vi "TestLocalize.vi"() -> ()   [LabVIEW 2011]
uses:
  JTrkAPI.llb/TrackerDLL.vi
panel:
  in  "Use QI":bool=TRUE
  in  "QI iterations":i32=2
  out "error":bool
  out "QI results":cluster{dbl, dbl}(graph)
  in  "ZLUT radius":sgl=32.0
  in  "profileWidth":i32=32
  out "ZLUT":sgl[][](graph)
  out "Intensity Graph":sgl[][](graph)
  in  "image size":cluster{"width":u32, "height":u32}={"width"=150, "height"=150}
  in  "Z random factor":dbl
  in  "z center":dbl=0.5
  out "Z localization":dbl(graph)
  in  "x scalefactor":sgl=0.1
  out "X Chart":dbl(graph)
  in  "jump period":i32=20
  in  "XCorWindow":u32=128
  in  "maxphotoncount":sgl=50000.0
  in  "Max Z":sgl=6.0
  in  "Min Z":sgl=1.0
  in  "Z planes":i32=60
  out "FPS":dbl
  out "Loop count":i32
  out "appended path":path
  in  "Show graphs":bool
  in  "Use debug library":bool
  in  "xcor_iterations":i32=2
  out "X profile":sgl[](graph)
  out "Y profile":sgl[](graph)
  out "Y result":sgl[](graph)
  out "True Y":dbl
  out "True X":dbl
  out "COM results":cluster{dbl, dbl}(graph)
  out "XCor results":cluster{dbl, dbl}(graph)
  in  "y center":dbl=75.0
  in  "x center":dbl=75.0 min=40.0 max=200.0
  out "X result":sgl[](graph)
  in  "Stop loop":bool
  out "median":sgl
  out "xcorpos":cluster{"XCor X":sgl, "XCor Y":sgl}
  out "COM":cluster{"comX":sgl, "comY":sgl}
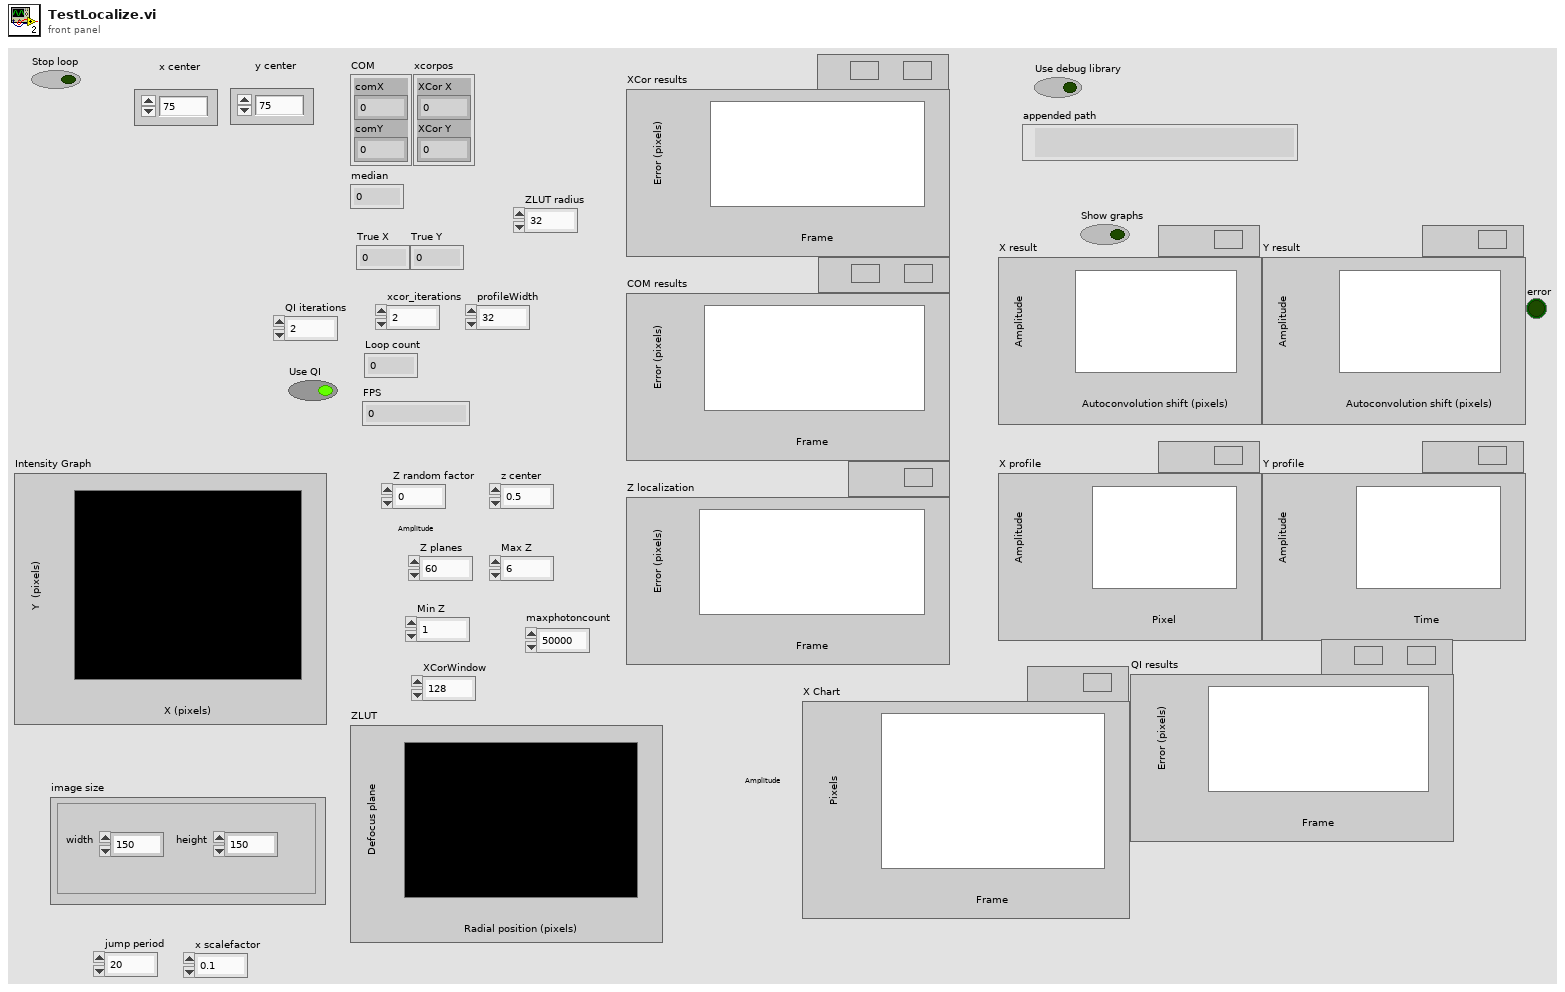
[diagram p1: front panel]
types:
  T1 = typedef "TrackerInstance.ctl" = cluster{"Tracker Pointer":u64, "Image size":cluster{"width":u32, "height":u32}}
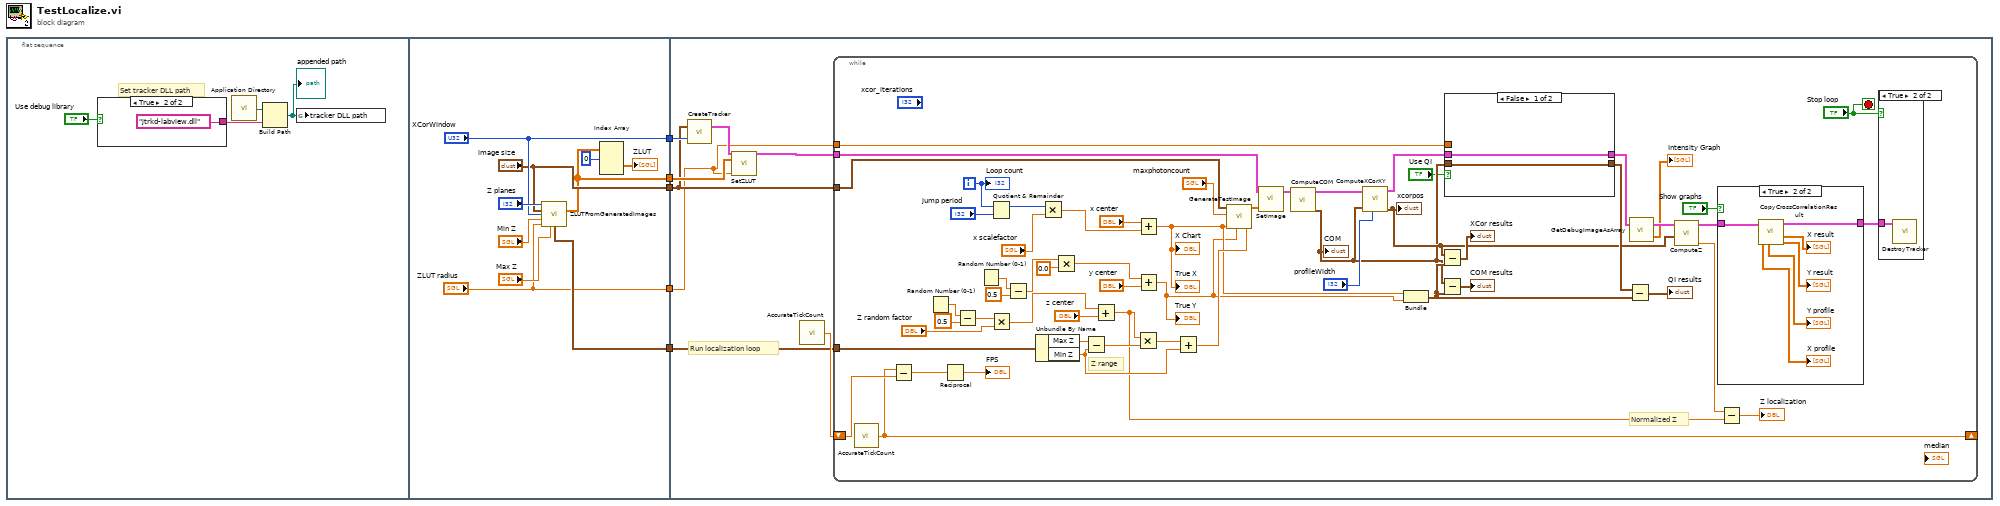
[diagram p0: block diagram]
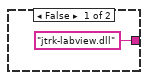
[diagram p2: hidden frame]
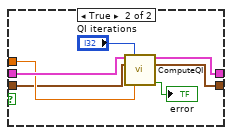
[diagram p3: hidden frame]
diagram:
  n1 = flat-sequence {
    tunnel: [w20] -> w5
    tunnel: ["image size"] -> w4
    tunnel: ["XCorWindow"] -> w3
    tunnel: [w13] -> w2
    tunnel: ["ZLUT radius"] -> w1
    tunnel: w5 -> [w28]
    tunnel: w4 -> [w25]
    tunnel: w3 -> [w27]
    tunnel: w2 -> [w26]
    tunnel: w1 -> [w22]
    frame #0 {
      # "Set tracker DLL path"
      n2 = case shown="True" "Use debug library" {
        tunnel: ["jtrk-labview.dll" "jtrkd-labview.dll"] -> w7
        frame False {
        }
        frame True {
        }
      }
      n3 = call <vilib>:"Application Directory.vi"() -> ("Application Directory"=w6:path)
      n4 = Build Path(base path=w6, name or relative path=w7) -> (appended path=w8:path)
      "appended path" <- w8
      n5 = global write "TrackerDLL.vi" "tracker DLL path"(w8) -> ()
    }
    frame #1 {
      n6 = call "ZLUTFromGeneratedImages.vi"("Z planes"="Z planes", "Image size"="image size", "XCorWindow"="XCorWindow", "Min Z"="Min Z", "maxradius"="ZLUT radius", "Max Z"="Max Z") -> ("ZLUT"=w13:sgl[][][], "z range"=w20:cluster{"Min Z":sgl, "Max Z":sgl})  [unwired: 8 in]
      n7 = Index Array(array=w13, index (dim 0)=0 ("index (page)")) -> (element=→"ZLUT":sgl[][])  [unwired: 2 in]
    }
    frame #2 {
      # "Run localization loop"
      n8 = call "CreateTracker.vi"("XCorWindow"=w27, "Image size"=w25) -> ("tracker"=w24:T1)  [unwired: 1 in]
      n9 = call "SetZLUT.vi"("tracker instance"=w24, "zluts"=w26, "maxradius"=w22) -> ("tracker"=w23:T1)  [unwired: 12 in]
      n10 = call "AccurateTickCount.vi"() -> ("seconds"=w29:dbl)
      n11 = while {
        tunnel: w23 -> [w32]
        shift-right: [w77] -> _
        shift-left: w29 -> [w78]
        tunnel: w25 -> [w74]
        tunnel: w28 -> [w62]
        tunnel: w22 -> [w39]
        i -> [w71]
        stop <- "Stop loop" stop-if-true
        # "Normalized Z"
        # "Z range"
        n12 = call "AccurateTickCount.vi"() -> ("seconds"=w77:dbl)
        n13 = Subtract(x=w77, y=w78) -> (x-y=w76:dbl)
        n14 = Random Number (0-1)() -> (number: 0 to 1=w64:dbl)
        n15 = Reciprocal(x=w76) -> (1/x=→"FPS":dbl)
        n16 = Subtract(x=w64, y=0.5) -> (x-y=w52:dbl)
        n17 = Random Number (0-1)() -> (number: 0 to 1=w83:dbl)
        n18 = Quotient & Remainder(x=w71, y="jump period") -> (x-y*floor(x/y)=w69:i32)  [unwired: 1 out]
        n19 = Multiply(x=w52, y="Z random factor") -> (x*y=w50:dbl)
        n20 = Subtract(x=w83, y=0.5) -> (x-y=w81:dbl)
        n21 = Unbundle By Name(w62) -> ("Max Z"=w61:sgl, "Min Z"=w58:sgl)
        n22 = Multiply(x=w69, y="x scalefactor") -> (x*y=w67:sgl)
        n23 = Multiply(x=w81, y=sgl 0.0) -> (x*y=w85:dbl)
        n24 = Subtract(x=w61, y=w58) -> (x-y=w59:sgl)
        n25 = Add(x=w50, y="z center") -> (x+y=w54:dbl)
        n26 = Multiply(x=w54, y=w59) -> (x*y=w57:dbl)
        n27 = Add(x="x center", y=w67) -> (x+y=w49:dbl)
        "True X" <- w49
        "X Chart" <- w49
        n28 = Add(x=w85, y="y center") -> (x+y=w48:dbl)
        "True Y" <- w48
        n29 = Add(x=w57, y=w58) -> (x+y=w56:dbl)
        n30 = call "GenerateTestImage.vi"("spotsize"=w56, "ypos"=w48, "xpos"=w49, "maxphotoncount"="maxphotoncount", "Image size"=w74) -> ("image"=w34:sgl[][])  [unwired: 4 in]
        n31 = call "SetImage.vi"("tracker"=w32, "Image (float)"=w34) -> ("tracker"=w33:T1)  [unwired: 6 in, 1 out]
        n32 = call "ComputeCOM.vi"("tracker"=w33) -> ("position"=w31:cluster{"X":sgl, "Y":sgl}, "tracker"=w43:T1)  [unwired: 5 in]
        "COM" <- w31
        n33 = call "ComputeXCorXY.vi"("tracker"=w43, "position"=w31, "profileWidth"="profileWidth") -> ("tracker"=w41:T1, "position"=w35:cluster{"X":sgl, "Y":sgl})  [unwired: 2 in, 2 out]
        "xcorpos" <- w35
        n34 = Bundle(w49, w48) -> (w36:cluster{dbl, dbl})  [unwired: 1 in]
        n35 = Subtract(x=w35, y=w36) -> (x-y=→"XCor results":cluster{dbl, dbl})
        n36 = Subtract(x=w31, y=w36) -> (x-y=→"COM results":cluster{dbl, dbl})
        n37 = case shown="False" "Use QI" {
          tunnel: w41 -> [w88 w95]
          tunnel: [w88 w94] -> w40
          tunnel: w39 -> [_ w93]
          tunnel: [w87 w92] -> w38
          tunnel: w31 -> [w87 w89]
          frame False {
          }
          frame True {
            n38 = call "ComputeQI.vi"("tracker"=w95, "iterations"="QI iterations", "initial position"=w89, "maxRadius"=w93) -> ("tracker"=w94:T1, "position"=w92:cluster{"X":sgl, "Y":sgl}, "error"=→"error":bool)  [unwired: 9 in]
          }
        }
        n39 = Subtract(x=w38, y=w36) -> (x-y=→"QI results":cluster{dbl, dbl})
        n40 = call "GetDebugImageAsArray.vi"("tracker"=w40) -> ("image"=→"Intensity Graph":sgl[][], "tracker"=w45:T1)  [unwired: 1 in]
        n41 = call "ComputeZ.vi"("position"=w35, "tracker instance"=w45) -> ("Z"=w55:sgl, "tracker instance"=w66:T1)  [unwired: 5 in, 2 out]
        n42 = case shown="True" "Show graphs" {
          tunnel: w66 -> [w96 w97]
          tunnel: [w96 w102] -> w80
          frame False {
          }
          frame True {
            n43 = call "CopyCrossCorrelationResult.vi"("tracker"=w97) -> ("x prof"=→"X profile":sgl[], "y prof"=→"Y profile":sgl[], "tracker"=w102:T1, "x result"=→"X result":sgl[], "y_result"=→"Y result":sgl[])  [unwired: 3 in]
          }
        }
        n44 = Subtract(x=w55, y=w54) -> (x-y=→"Z localization":dbl)
        n45 = case shown="True" "Stop loop" {
          tunnel: w80 -> [_ w103]
          frame False {
          }
          frame True {
            n46 = call "DestroyTracker.vi"("tracker instance"=w103) -> ()  [unwired: 5 in]
          }
        }
        "Loop count" <- w71
      }
    }
  }
